vi "温度采集初始化.vi"(8 "错误输入（无错误）":errorcluster, 10 "温度探头":string, 11 "VISA资源名称":refnum<visa-resource-name>) -> (0 "error out":errorcluster caption="错误输出", 3 "DMM 输出":refnum<class "DMM.lvclass">)   [LabVIEW 2021]
uses:
  DMM/DMM.lvclass
  <vilib>/regexp/Match Regular Expression.xnode
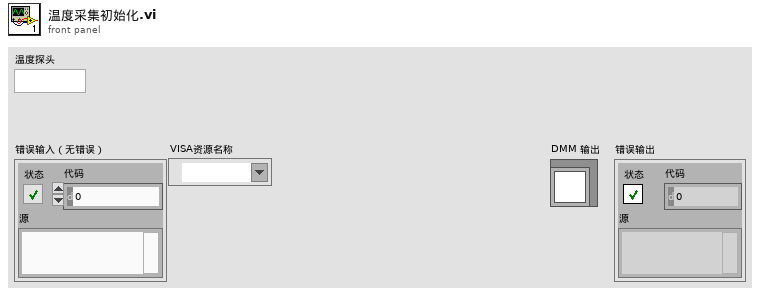
[diagram p1: front panel]
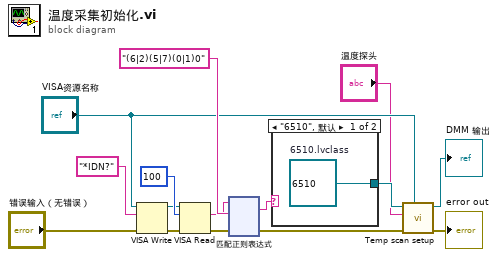
[diagram p0: block diagram]
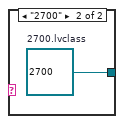
[diagram p2: hidden frame]
diagram:
  n1 = VISA Write(VISA resource name="VISA资源名称", write buffer="*IDN?" ("写入缓冲区"), error in (no error)="错误输入（无错误）") -> (VISA resource name out=w2:refnum<visa-resource-name>, error out=w14:errorcluster)  [unwired: 1 out]
  n2 = VISA Read(VISA resource name=w2, byte count=u32 100 ("字节总数"), error in (no error)=w14) -> (read buffer=w11:string, error out=w10:errorcluster)  [unwired: 2 out]
  n3 = xnode "匹配正则表达式"("输入字符串"=w11, "正则表达式"="(6|2)(5|7)(0|1)0", "错误输入"=w10) -> ("所有匹配"=w8:string, "错误输出"=w5:errorcluster)  [unwired: 3 in, 3 out]
  n4 = case shown="\"6510\", 默认" w8 {
    tunnel: [w16 w17] -> w7
    frame "6510", Default {
      w16 = refnum<class "6510.lvclass"> refnum  # 6510.lvclass
    }
    frame "2700" {
      w17 = refnum<class "2700.lvclass"> refnum  # 2700.lvclass
    }
  }
  n5 = call-dynamic "Temp scan setup.vi"("VISA资源名称"="VISA资源名称", "error in (no error)"=w5, "字符串"="温度探头", "DMM 输入"=w7) -> ("error out"=→"error out":errorcluster, "DMM 输出"=→"DMM 输出":refnum<class "DMM.lvclass">)  [unwired: 6 in]
